vi "VI Refname.vi"(8 "error in (no error)":errorcluster, 10 "VI in":refnum<vi>, 11 "ViName":string) -> (0 "error out":errorcluster, 2 "VI out":refnum<vi>, 3 "Name":string)   [LabVIEW 2017, in "TagDB RefManager.lvlib"]
uses:
  TagDB RefManager.lvlib
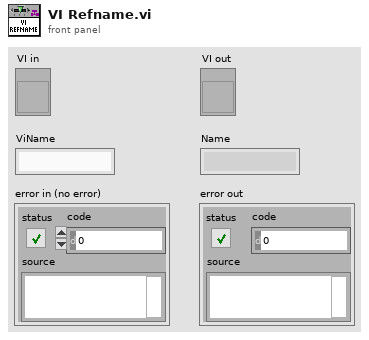
[diagram p1: front panel]
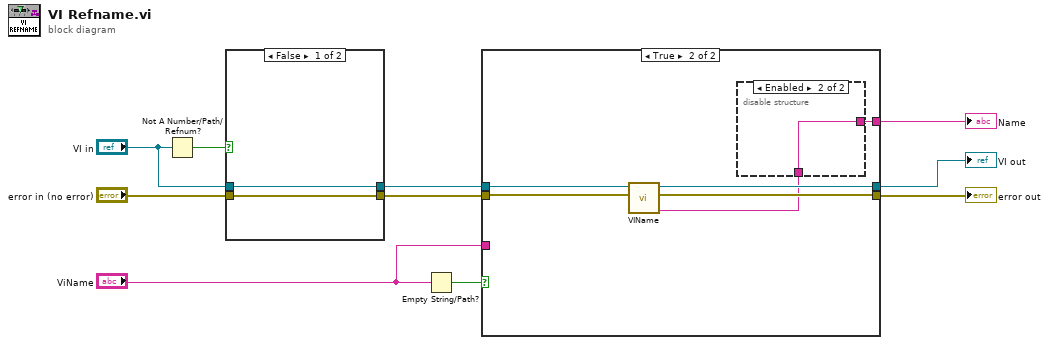
[diagram p0: block diagram]
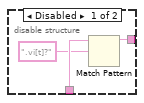
[diagram p3: hidden frame]
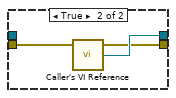
[diagram p4: hidden frame]
diagram:
  n1 = Not A Number/Path/Refnum?(number/path/refnum="VI in") -> (NaN/Path/Refnum?=w7:bool)
  n2 = case shown="False" w7 {
    tunnel: "VI in" -> [w12 _]
    tunnel: [w12 w15] -> w2
    tunnel: "error in (no error)" -> [w11 w13]
    tunnel: [w11 w14] -> w9
    frame False {
    }
    frame True {
      n3 = call "Caller's VI Reference.vi"("error in (no error)"=w13) -> ("error out"=w14:errorcluster, "Caller's VI Reference"=w15:refnum<vi>)  [unwired: 5 in]
    }
  }
  n4 = Empty String/Path?(string/path="ViName") -> (empty?=w3:bool)
  n5 = case shown="True" w3 {
    tunnel: w2 -> [w17 w22]
    tunnel: [w17 w24] -> w6
    tunnel: w9 -> [w16 w21]
    tunnel: [w16 w20] -> w5
    tunnel: [w18 w23] -> w10
    tunnel: "ViName" -> [w18 _]
    frame False {
    }
    frame True {
      n6 = call "VIName.vi"("error in (no error)"=w21, "VI in"=w22) -> ("Name"=w19:string, "error out"=w20:errorcluster, "VI out"=w24:refnum<vi>)  [unwired: 7 in]
      n7 = disable-structure shown="Enabled" {
        disable-tunnel: w19 -> [w27 w28]
        disable-tunnel: [w26 w28] -> w23
        frame Disabled {
          n8 = Match Pattern(string=w27, regular expression=".vi[t]?") -> (before substring=w26:string)  [unwired: 1 in, 3 out]
        }
        frame Enabled {
        }
      }
    }
  }
  "Name" <- w10
  "VI out" <- w6
  "error out" <- w5
